vi "未命名 3.vi"() -> ()   [LabVIEW 2011, in "List.lvlib"]
uses:
  List.lvlib
  List/List.lvclass
  DATA.lvclass
panel:
  out "数值 2":dbl
  out "名称 2":string
  out "数值":dbl
  out "名称":string
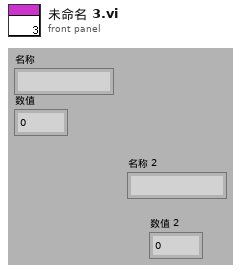
[diagram p1: front panel]
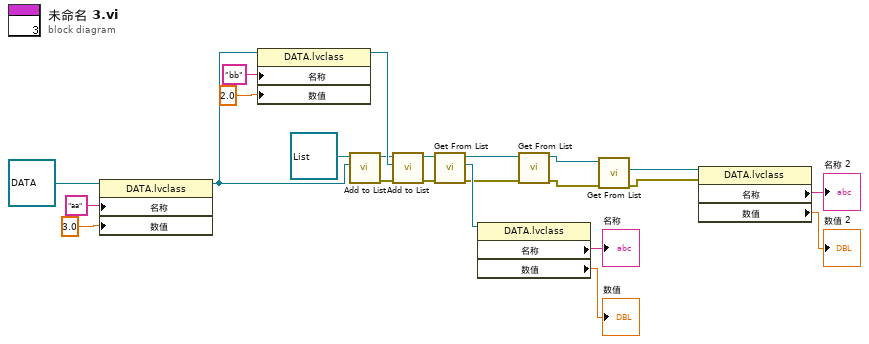
[diagram p0: block diagram]
diagram:
  n1 = property class="DATA.lvclass"(reference=refnum<class "DATA.lvclass"> refnum ("List.lvlib:DATA.lvclass"), "名称"="aa", "数值"=3.0) -> (reference out=w19:refnum<class "DATA.lvclass">)  [unwired: 1 in, 1 out]
  n2 = property class="DATA.lvclass"(reference=w19, "名称"="bb", "数值"=2.0) -> (reference out=w16:refnum<class "DATA.lvclass">)  [unwired: 1 in, 1 out]
  n3 = call "Add to List.vi"("List.lvlib:DATA.lvclass"=w19, "List 输入"=refnum<class "List.lvclass"> refnum ("List.lvlib:List.lvclass")) -> ("error out"=w14:errorcluster, "List 输出"=w15:refnum<class "List.lvclass">)  [unwired: 8 in]
  n4 = call "Add to List.vi"("error in (no error)"=w14, "List.lvlib:DATA.lvclass"=w16, "List 输入"=w15) -> ("error out"=w12:errorcluster, "List 输出"=w13:refnum<class "List.lvclass">)  [unwired: 7 in]
  n5 = call "Get From List.vi"("error in (no error)"=w12, "List 输入"=w13) -> ("error out"=w8:errorcluster, "List.lvlib:DATA.lvclass"=w11:refnum<class "DATA.lvclass">, "List 输出"=w7:refnum<class "List.lvclass">)  [unwired: 7 in]
  n6 = property class="DATA.lvclass"(reference=w11) -> ("名称"=→"名称":string, "数值"=→"数值":dbl)  [unwired: 1 in, 2 out]
  n7 = call "Get From List.vi"("error in (no error)"=w8, "List 输入"=w7) -> ("error out"=w4:errorcluster, "List 输出"=w3:refnum<class "List.lvclass">)  [unwired: 7 in, 1 out]
  n8 = call "Get From List.vi"("error in (no error)"=w4, "List 输入"=w3) -> ("error out"=w2:errorcluster, "List.lvlib:DATA.lvclass"=w1:refnum<class "DATA.lvclass">)  [unwired: 7 in, 1 out]
  n9 = property class="DATA.lvclass"(reference=w1, error in=w2) -> ("名称"=→"名称 2":string, "数值"=→"数值 2":dbl)  [unwired: 2 out]
